vi "repeat cycle_normal.vi"(8 "error in (no error)":errorcluster caption="에러 입력(에러 없음)", 10 "waveform in":waveform(dbl), 11 "Waveform Obj 입력":refnum<class "PWL_DW7802.lvclass">) -> (0 "error out":errorcluster caption="에러 출력", 2 "waveform out":waveform(dbl), 3 "Waveform Obj 출력":refnum<class "PWL_DW7802.lvclass">)   [LabVIEW 2020, in "PWL_DW7802.lvclass"]
uses:
  PWL_DW7802.lvclass
  Waveform Gen/Waveform Gen.lvclass/Waveform Gen.ctl
  Waveform Gen/Accessors/Read scale.vi
  PWL/PWL.lvclass
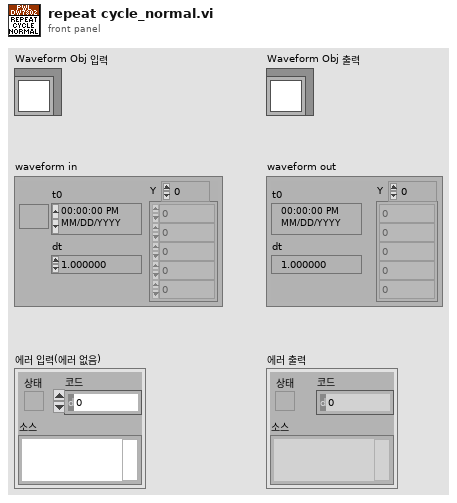
[diagram p1: front panel]
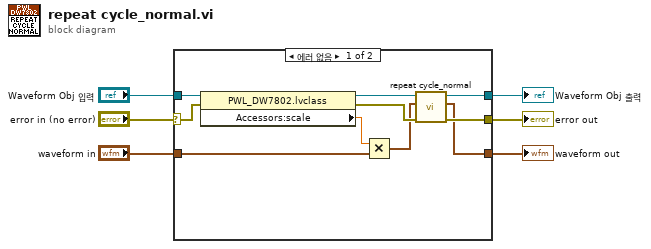
[diagram p0: block diagram]
diagram:
  n1 = case shown="에러 없음" "error in (no error)" {
    selector: "error in (no error)" -> [w14 w18]
    tunnel: [w16 w19] -> w6
    tunnel: "Waveform Obj 입력" -> [w11 w19]
    tunnel: [w15 w18] -> w4
    tunnel: [w13 w17] -> w2
    tunnel: "waveform in" -> [w8 w17]
    frame No Error {
      n2 = property class="PWL_DW7802.lvclass"(reference=w11, error in=w14) -> (reference out=w10:refnum<class "PWL_DW7802.lvclass">, error out=w12:errorcluster, "Accessors:scale"=w9:dbl)
      n3 = Multiply(x=w9, y=w8) -> (x*y=w7:waveform(dbl))
      n4 = call-parent "repeat cycle_normal.vi"("error in (no error)"=w12, "waveform in"=w7, "Waveform Obj 입력"=w10) -> ("error out"=w15:errorcluster, "waveform out"=w13:waveform(dbl), "Waveform Obj 출력"=w16:refnum<class "PWL_DW7802.lvclass">)  [unwired: 6 in]
    }
    frame Error {
    }
  }
  "error out" <- w4
  "Waveform Obj 출력" <- w6
  "waveform out" <- w2
